vi "dfd_Validate Params for One Point Notch Peak Design by BW.vi"(6 "fs [Hz]":dbl=1.0 format="%.2f", 8 "error in (no error)":errorcluster, 9 "bandwidth":dbl=35.0 format="%.2f", 10 "Ab [dB]":dbl=3.0 format="%.2f", 11 "f0 [Hz]":dbl format="%.2f") -> (0 "error out":errorcluster, 1 "normalized bandwidth":dbl format="%.2f", 2 "dup Ab [dB]":dbl format="%.2f", 3 "normalized f0":dbl format="%.2f")   [LabVIEW 2017, in "NI_DigFilter_Design.lvlib"]
uses:
  <vilib>/addons/Digital Filter Design/NI_DigFilter_Design.lvlib
  <vilib>/addons/Digital Filter Design/_Misc.llb/dfd_Error Handlers (Multiple).vi
  <vilib>/addons/Digital Filter Design/NI_DigFilterLicensed.lvlib
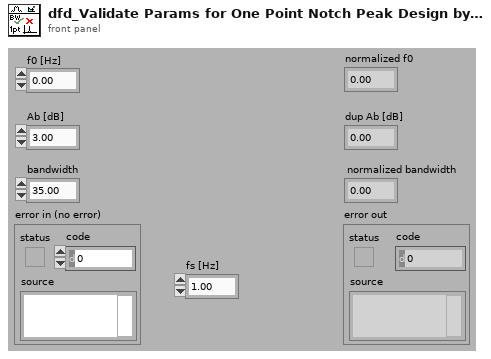
[diagram p1: front panel]
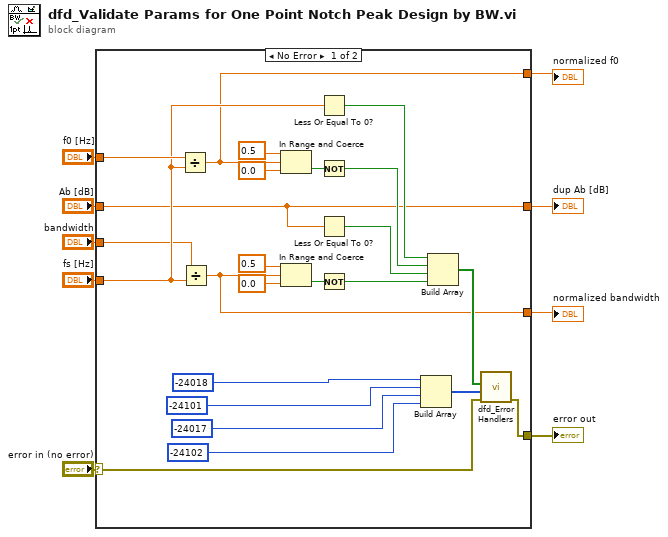
[diagram p0: block diagram]
diagram:
  n1 = case shown="No Error" "error in (no error)" {
    selector: "error in (no error)" -> [w31 w34]
    tunnel: [w11 _] -> w9
    tunnel: "Ab [dB]" -> [w11 _]
    tunnel: "bandwidth" -> [w10 _]
    tunnel: "f0 [Hz]" -> [w33 _]
    tunnel: [w32 w34] -> w5
    tunnel: "fs [Hz]" -> [w28 _]
    tunnel: [w26 _] -> w3
    tunnel: [w20 _] -> w2
    frame No Error {
      n2 = Divide(x=w33, y=w28) -> (x/y=w26:dbl)
      n3 = Divide(x=w10, y=w28) -> (x/y=w20:dbl)
      n4 = In Range and Coerce(upper limit=0.5 ("y"), x=w26, lower limit=0.0 ("y")) -> (In Range?=w24:bool)  [unwired: 1 out]
      n5 = In Range and Coerce(upper limit=0.5 ("y"), x=w20, lower limit=0.0 ("y")) -> (In Range?=w21:bool)  [unwired: 1 out]
      n6 = Less Or Equal To 0?(x=w28) -> (x <= 0?=w19:bool)
      n7 = Not(x=w24) -> (.not. x?=w18:bool)
      n8 = Less Or Equal To 0?(x=w11) -> (x <= 0?=w14:bool)
      n9 = Not(x=w21) -> (.not. x?=w15:bool)
      n10 = Build Array(-24018 ("ERR_FS_LE_ZERO"), -24101 ("ERR_F0BYBW_RANGE_WRONG"), -24017 ("ERR_dB_LE_ZERO"), -24102 ("ERR_BW_RANGE_WRONG")) -> (w29:i32[])
      n11 = Build Array(w19, w18, w14, w15) -> (w30:bool[])
      n12 = call-poly <vilib>:"dfd_Error Handlers.vi"("error in (no error)"=w31, "error sources"=w29, "condition failed?"=w30) -> ("error out"=w32:errorcluster)  [unwired: 8 out]
    }
    frame Error {
    }
  }
  "dup Ab [dB]" <- w9
  "normalized bandwidth" <- w2
  "normalized f0" <- w3
  "error out" <- w5
